vi "TCP Timing Test.vi"() -> ()   [LabVIEW 2015]
uses:
  <vilib>/Analysis/baseanly.llb/Mean (DBL).vi
  <vilib>/Analysis/NI_AALBase.lvlib
panel:
  out "Waveform Graph":u32[](graph)
  out "Numeric":i32
  out "mean":dbl format="%0.2f"
  out "min value":u32
  out "max value":u32
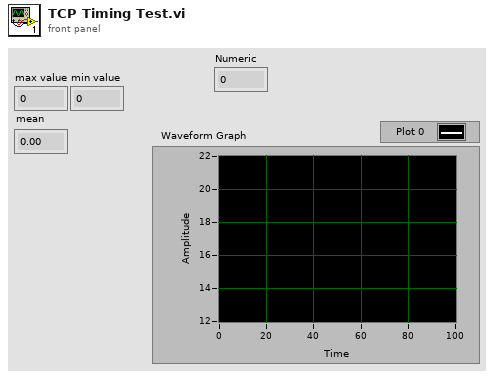
[diagram p1: front panel]
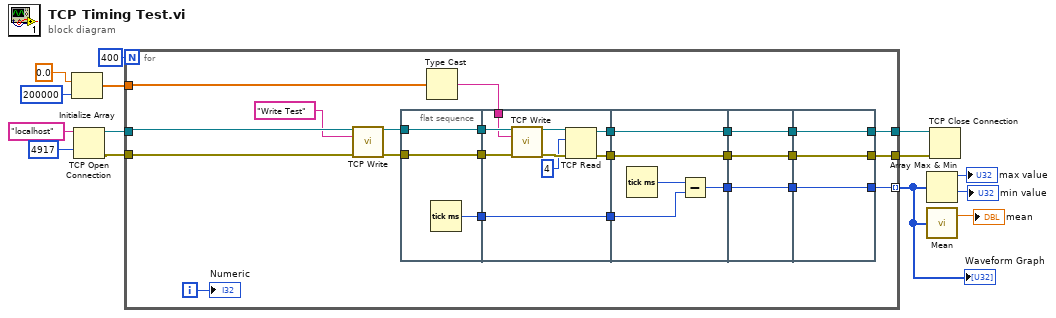
[diagram p0: block diagram]
diagram:
  n1 = Initialize Array(0.0 ("element"), 200000 ("dimension size")) -> (w11:dbl[])
  n2 = TCP Open Connection(address="localhost", remote port or service name=u16 4917) -> (connection ID=w5:refnum<k5>, error out=w4:errorcluster)  [unwired: 3 in]
  n3 = for {
    N: 400 -> [_]
    tunnel: w11 -> [w35]
    tunnel: [w31] -> w1 mode=indexing
    tunnel: w5 -> [w16]
    tunnel: w4 -> [w19]
    tunnel: [w23] -> w3
    tunnel: [w21] -> w2
    i -> [w28]
    n4 = call "TCP Write.vi"("connection ID"=w16, "data string"="Write Test" ("address"), "error in (no error)"=w19) -> ("connection ID out"=w17:refnum<k5>, "error out"=w18:errorcluster)  [unwired: 10 in, 1 out]
    n5 = flat-sequence {
      tunnel: w17 -> [w39]
      tunnel: w18 -> [w40]
      tunnel: [w40] -> w37
      tunnel: [w39] -> w36
      tunnel: [w38] -> w33
      tunnel: w37 -> [w45]
      tunnel: w36 -> [w46]
      tunnel: w34 -> [w41]
      tunnel: w33 -> [w49]
      tunnel: [w49] -> w32
      tunnel: [w48] -> w30
      tunnel: [w47] -> w29
      tunnel: w32 -> [w53]
      tunnel: w30 -> [w50]
      tunnel: w29 -> [w51]
      tunnel: [w52] -> w27
      tunnel: [w51] -> w26
      tunnel: [w50] -> w25
      tunnel: w27 -> [w57]
      tunnel: w26 -> [w55]
      tunnel: w25 -> [w56]
      tunnel: [w57] -> w24
      tunnel: [w56] -> w22
      tunnel: [w55] -> w20
      tunnel: [w60] -> w31
      tunnel: w24 -> [w60]
      tunnel: [w59] -> w23
      tunnel: w22 -> [w59]
      tunnel: [w58] -> w21
      tunnel: w20 -> [w58]
      frame #0 {
        n6 = Tick Count (ms)() -> (millisecond timer value=w38:u32)
      }
      frame #1 {
        n7 = call "TCP Write.vi"("connection ID"=w46, "data string"=w41, "error in (no error)"=w45) -> ("connection ID out"=w42:refnum<k5>, "error out"=w44:errorcluster)  [unwired: 10 in, 1 out]
        n8 = TCP Read(connection ID=w42, bytes to read=4, error in (no error)=w44) -> (connection ID out=w47:refnum<k5>, error out=w48:errorcluster)  [unwired: 2 in, 1 out]
      }
      frame #2 {
        n9 = Tick Count (ms)() -> (millisecond timer value=w54:u32)
        n10 = Subtract(x=w54, y=w53) -> (x-y=w52:u32)
      }
      frame #3 {
      }
      frame #4 {
      }
    }
    n11 = Type Cast(x=w35) -> (*(type *) &x=w34:string)  [unwired: 1 in]
    "Numeric" <- w28
  }
  "Waveform Graph" <- w1
  n12 = Array Max & Min(array=w1) -> (max value=→"max value":u32, min value=→"min value":u32)  [unwired: 2 out]
  n13 = call-poly <vilib>:"Mean.vi"("X"=w1) -> ("mean"=→"mean":dbl)  [unwired: 1 out]
  n14 = TCP Close Connection(connection ID=w2, error in (no error)=w3) -> ()  [unwired: 1 in, 2 out]
